vi "Get BLISS_Choose next server list.vi"(10 "Server List by Status":T1) -> (3 "Updated Server List":string[](array[string]))   [LabVIEW 2020]
uses:
  Get BLISS_Server List by Status.ctl
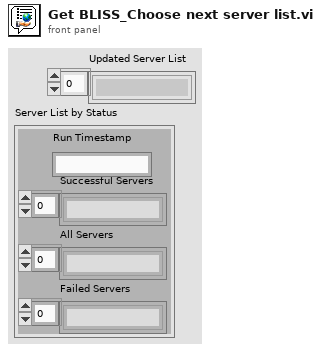
[diagram p1: front panel]
types:
  T1 = typedef "Get BLISS_Server List by Status.ctl" = cluster{"Successful Servers":string[], "All Servers":string[], "Failed Servers":string[], "Run Timestamp":string}
  T2 = enum16{"Left Button", "Center Button", "Right Button", "Window Close"}
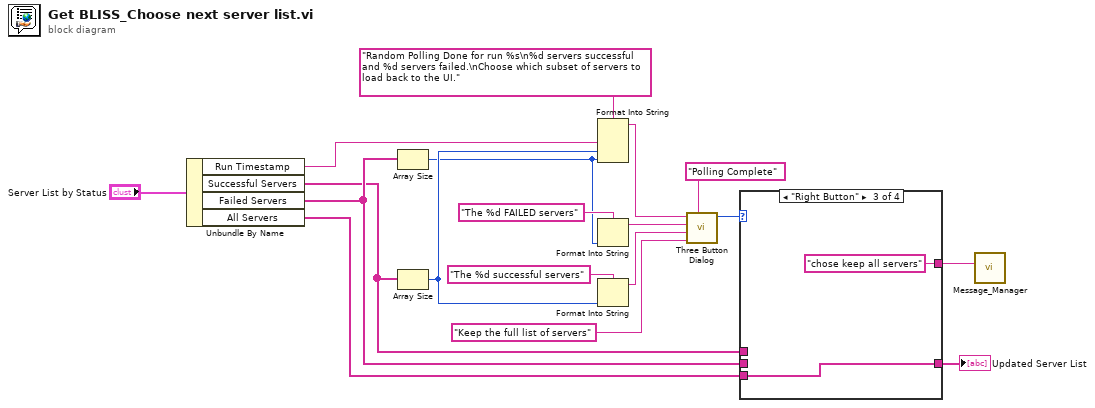
[diagram p0: block diagram]
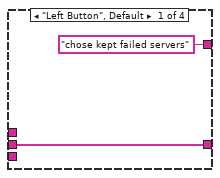
[diagram p2: hidden frame]
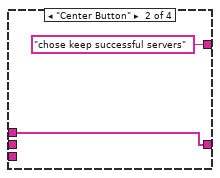
[diagram p3: hidden frame]
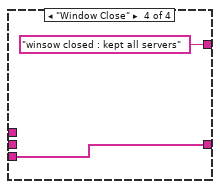
[diagram p4: hidden frame]
diagram:
  n1 = Unbundle By Name("Server List by Status") -> ("Run Timestamp"=w1:string, "Successful Servers"=w5:string[], "Failed Servers"=w6:string[], "All Servers"=w7:string[])
  n2 = Array Size(array=w6) -> (size(s)=w3:i32)
  n3 = Array Size(array=w5) -> (size(s)=w4:i32)
  n4 = Format Into String(format string="Random Polling Done for run %s\n%d servers successful and %d servers failed.\nChoose which subset of servers to load back to the UI." ("message"), w1, w4, w3) -> (resulting string=w18:string)  [unwired: 2 in, 1 out]
  n5 = Format Into String(format string="The %d FAILED servers" ("Left Button Text (\"Yes\")"), w3) -> (resulting string=w13:string)  [unwired: 2 in, 1 out]
  n6 = Format Into String(format string="The %d successful servers" ("Left Button Text (\"Yes\")"), w4) -> (resulting string=w14:string)  [unwired: 2 in, 1 out]
  n7 = call <vilib>:"Three Button Dialog.vi"("Window Title (\"\")"="Polling Complete" ("Window Title (\"\")"), "Right Button Text (\"Cancel\")"="Keep the full list of servers" ("Left Button Text (\"Yes\")"), "Center Button Text (\"No\")"=w14, "Left Button Text (\"Yes\")"=w13, "message"=w18) -> ("Which Button?"=w12:T2)  [unwired: 6 in]
  n8 = case shown="\"Right Button\"" w12 {
    tunnel: [w20 w22 w24 w26] -> w16
    tunnel: w6 -> [w20 _ _ _]
    tunnel: w5 -> [_ w22 _ _]
    tunnel: w7 -> [_ _ w24 w26]
    tunnel: ["chose kept failed servers" ("New Entry") "chose keep successful servers" ("New Entry") "chose keep all servers" ("New Entry") "winsow closed : kept all servers" ("New Entry")] -> w2
    frame "Left Button", Default {
    }
    frame "Center Button" {
    }
    frame "Right Button" {
    }
    frame "Window Close" {
    }
  }
  "Updated Server List" <- w16
  n9 = call "Message_Manager.vi"("New Entry"=w2) -> ()  [unwired: 5 in, 6 out]
